vi "Shutdown.vi"(8 "error in (no error)":errorcluster, 11 "JKI_Python_Server in":refnum<class "Server.lvclass">) -> (0 "error out":errorcluster)   [LabVIEW 2013, in "JKI_Python_Bridge_for_LV.lvlib" / "Server.lvclass"]
uses:
  Server.lvclass
  Server.lvclass/Server.ctl
  CallHandler/PyObject.lvclass/PyObject.ctl
  CallHandler/PyObject.lvclass
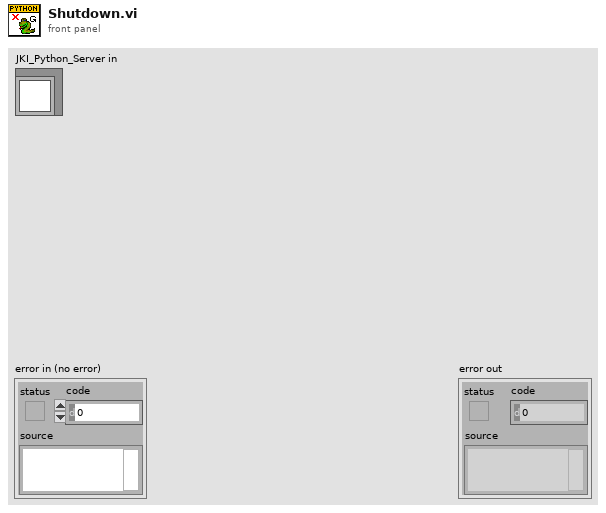
[diagram p1: front panel]
types:
  T1 = typedef "JKI_Python_Bridge_for_LV.lvlib/Server.lvclass/Class Private Data - Cluster.ctl" = cluster{"TCP Server RefNum":T2, "TCP port (50007)":u16, "max connections (0: no limit)":u32, "net address (0: Listen on All Adaptors)":u32, "Nodes":T3[], "Public Events":T4}
  T2 = typedef "TCP Server Object RefNum__jki_lib_tcp_server.ctl" = refnum<k1>
  T3 = typedef "JKI_Python_Bridge_for_LV.lvlib/Server.lvclass/Python Node.ctl" = cluster{"Name":string, "Python Method Call":refnum<user-event>, "Call Handle":refnum<class "PyObject.lvclass">}
  T4 = typedef "JKI_Python_Bridge_for_LV.lvlib/Server.lvclass/Public Events - Cluster.ctl" = cluster{"Stop Nodes":refnum<user-event>}
  T5 = typedef "JKI_Python_Bridge_for_LV.lvlib/Server.lvclass/Python Method Call - Event Registration.ctl" = refnum<event-registration>
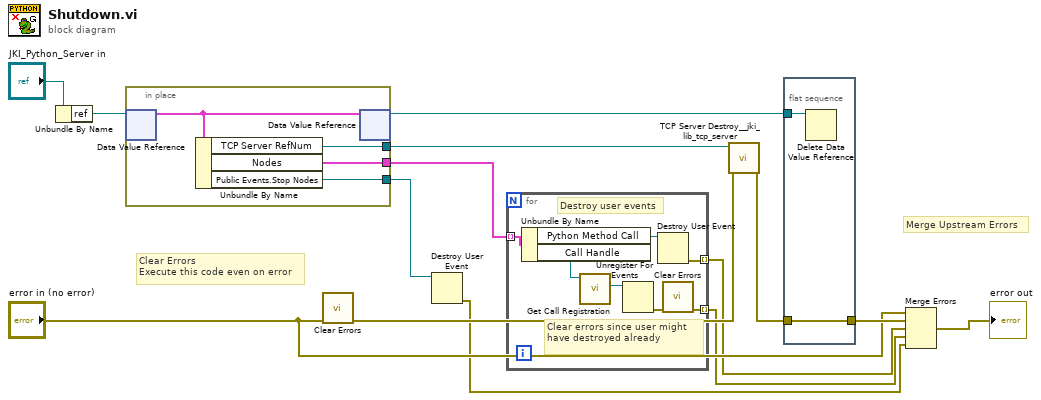
[diagram p0: block diagram]
diagram:
  # "Merge Upstream Errors"
  # "Clear Errors\nExecute this code even on error"
  n1 = Unbundle By Name("JKI_Python_Server in") -> ("ref"=w7:refnum<data-value>)
  n2 = in-place {
    in-place-border: [w18] -> w13
    in-place-border: [w16] -> w5
    in-place-border: [w15] -> w3
    n3 = in-place-dvr #1(w7) -> (w17:T1)  [unwired: 1 out]
    n4 = Unbundle By Name(w17) -> ("TCP Server RefNum"=w18:T2, "Nodes"=w16:T3[], "Public Events.Stop Nodes"=w15:refnum<user-event>)
    n5 = in-place-dvr #1(w17) -> (w6:refnum<data-value>)  [unwired: 1 out]
  }
  n6 = call <vilib>:"Clear Errors.vi"("error in (no error)"="error in (no error)") -> ("error out"=w11:errorcluster)  [unwired: 6 in]
  n7 = Destroy User Event(user event=w3) -> (error out=w2:errorcluster)  [unwired: 1 in]
  n8 = for {
    tunnel: w5 -> [w25] mode=indexing
    tunnel: [w23] -> w4 mode=indexing
    tunnel: [w19] -> w1 mode=indexing
    # "Clear errors since user might have destroyed already"
    # "Destroy user events"
    n9 = Unbundle By Name(w25) -> ("Python Method Call"=w24:refnum<user-event>, "Call Handle"=w22:refnum<class "PyObject.lvclass">)
    n10 = call "Get Call Registration.vi"("Node in"=w22) -> ("Call Registration"=w21:T5)  [unwired: 8 in, 2 out]
    n11 = Unregister For Events(event registration refnum=w21) -> (error out=w20:errorcluster)  [unwired: 1 in]
    n12 = Destroy User Event(user event=w24) -> (error out=w23:errorcluster)  [unwired: 1 in]
    n13 = call <vilib>:"Clear Errors.vi"("error in (no error)"=w20) -> ("error out"=w19:errorcluster)  [unwired: 6 in]
  }
  n14 = call <vilib>:"TCP Server Destroy__jki_lib_tcp_server.vi"("error in (no error)"=w11, "Object RefNum"=w13) -> ("error out"=w12:errorcluster)  [unwired: 9 out]
  n15 = flat-sequence {
    tunnel: [w27] -> w14
    tunnel: w12 -> [w27]
    tunnel: w6 -> [w26]
    frame #0 {
      n16 = Delete Data Value Reference(data value reference=w26) -> ()  [unwired: 1 in, 2 out]
    }
  }
  n17 = Merge Errors("error in (no error)", w14, w4, w1, w2) -> (→"error out":errorcluster)
